vi "Get Send Type.vi"(11 "Abstract Message Scripter in":refnum<class "Abstract Message Scripter.lvclass">) -> (2 "Send Type":enum16{"Concrete", "Abstract"}(ring))   [LabVIEW 2020, in "Message Maker.lvlib" / "Abstract Message Scripter.lvclass"]
uses:
  Abstract Message Scripter.lvclass
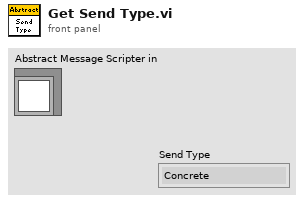
[diagram p1: front panel]
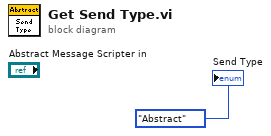
[diagram p0: block diagram]
diagram:
  "Send Type" <- enum16{"Concrete", "Abstract"}."Abstract" ("Send Type")
